vi "MrClean.ProcDestructor.vi"(0 "i ref in":refnum<vi>, 3 "ms timeout (100)":i32=100, 5 "error in (no error)":errorcluster) -> (14 "i ref out":refnum<vi>, 17 "timed out":bool, 19 "error out":errorcluster)   [LabVIEW 2014, in "MrClean.lvlib"]
doc: "This is the counterpart to ProcConstructor and is called befor the \"deactivate\" is called. This can be used to shutdown/deinitialize things."
uses:
  MrClean.lvlib
  CSCore/CSSystem/CoreDefs/CoreDefs.error_type.ctl
  CSCore/CSSystem/CoreLib/CoreLib.string 2 byte array.vi
  CSCore/BaseProcess/BaseProcess.lvlib
  LEBITLib/LEBITLib.lvlib
  CSCore/CSSystem/CSSystemLib/CSSystemLib.lvlib
  CSCore/CSSystem/CoreLib/CoreLib.lvlib
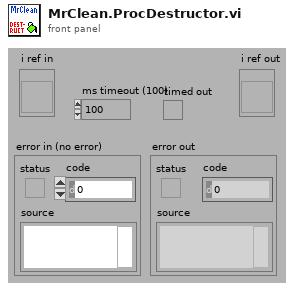
[diagram p1: front panel]
types:
  T1 = typedef "CoreDefs.error_type.ctl" = enum16{"no error", "can't load process", "can't unload process", "process does not exist", "can't install process", "can't remove process", "unknown function", "time out", "can't execute function", "duplicate queue name", "super not found", "caller queue invalid", "can't ping process", "unknown error", "VISA Error", "VISA timeout", "GPIB timeout", "GPIB error", "communication error", "data type mismatch", "can't read data from OPC server", "can't write data to OPC server", "OET error", "function not implemented", "process already exists", "invalid Shared Variable name", "error writing Shared Variable", "error reading Shared Variable", "invalid client name", "corrupt database", "unknown class", "call not authorized", "parameter out of range", "OET timeout: can't get data to modify", "invalid queue name", "requested operation incompatible with current state", "event undefined", "event disabled", "state undefined", "caller is not a friend", "EventBuilder: bad eventID", "EventBuilder: no DAQ devices", "a thread must not stop itself", "UNUSED ELEMENT4", "DiscArchiver: eventData incomplete", "DiscArchiver: eventData does not belong to run", "DiscArchiver: can't open file", "DiscArchiver: can't write to file", "DiscArchiver: available disc space low", "can't acquire semaphore", "error reading data from database", "notifier object is not existing", "can't register process", "can't unregister process", "illegal event type", "object disabled", "object already exists", "can't change state", "Instrument not found", "no connection to remote node", "invalid reference", "N/A", "UNUSED ELEMENT 1", "element not found", "illegal TCP/IP connection detected", "object does not exist", "invalid access ID", "unknown CS system", "invalid privilige", "unsupported data type", "unsupported server type", "IO server already exists", "Shared Variable already exists"}
  T2 = enum16{"simple", "synchronous", "asynchronous", "notification"}
  T3 = typedef "CoreDefs.rawDataType.ctl" = i8[]
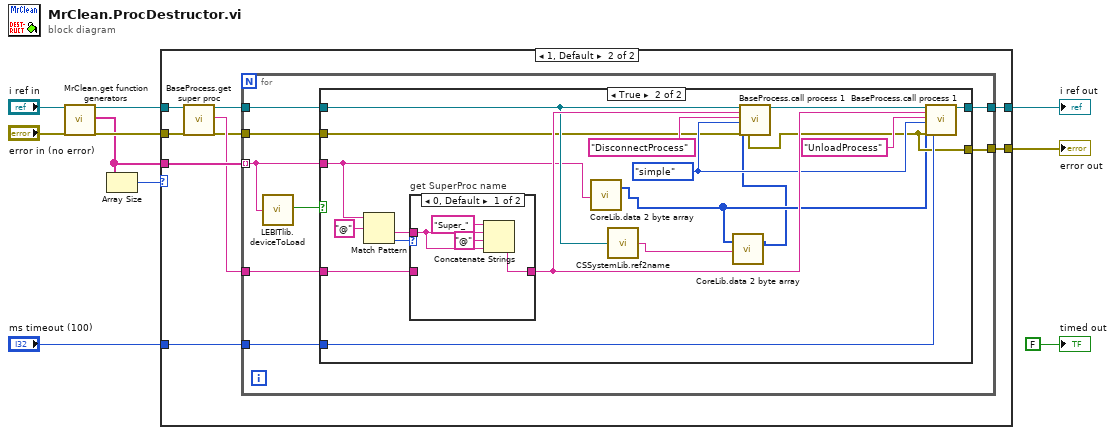
[diagram p0: block diagram]
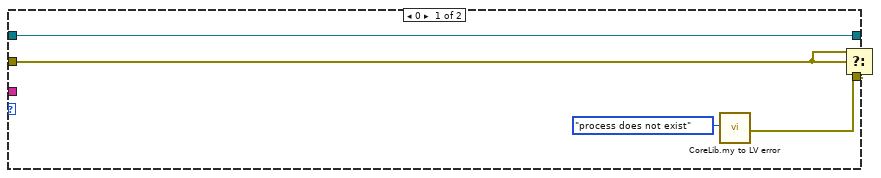
[diagram p2: hidden frame]
diagram:
  n1 = call "MrClean.get function generators.vi"("i ref in"="i ref in", "error in (no error)"="error in (no error)") -> ("i ref out"=w9:refnum<vi>, "function generators"=w7:string[], "error out"=w8:errorcluster)  [unwired: 14 in, 1 out]
  n2 = Array Size(array=w7) -> (size(s)=w10:i32)
  n3 = case shown="1, Default" w10 {
    tunnel: w9 -> [w15 w24]
    tunnel: w8 -> [w13 w23]
    tunnel: w7 -> [_ w21]
    tunnel: "ms timeout (100)" -> [_ w19]
    tunnel: [w14 w16] -> w1
    tunnel: [w15 w18] -> w2
    frame 0 {
      n4 = call "CoreLib.my to LV error.vi"("ErrorTypes"=CoreDefs.error_type."process does not exist") -> ("myErrorCluster"=w12:errorcluster)  [unwired: 17 in, 1 out]
      n5 = Select(t=w13, s=w13, f=w12) -> (s? t:f=w14:errorcluster)
    }
    frame 1, Default {
      n6 = call "BaseProcess.get super proc.vi"("i ref in"=w24, "error in (no error)"=w23) -> ("i ref out"=w22:refnum<vi>, "SuperProc"=w20:string, "error out"=w17:errorcluster)  [unwired: 15 in]
      n7 = for {
        tunnel: w22 -> [w29]
        tunnel: w21 -> [w25] mode=indexing
        tunnel: w20 -> [w32]
        tunnel: w19 -> [w30]
        tunnel: [w31] -> w18
        tunnel: w17 -> [w27]
        tunnel: [w28] -> w16
        n8 = call "LEBITlib.deviceToLoad.vi"("DeviceName"=w25) -> ("DeviceIsToLoad"=w26:bool)
        n9 = case shown="True" w26 {
          tunnel: w32 -> [_ w48]
          tunnel: w25 -> [_ w38]
          tunnel: [w33 w43] -> w31
          tunnel: w30 -> [_ w42]
          tunnel: w29 -> [w33 w40]
          tunnel: w27 -> [w34 w39]
          tunnel: [w34 w39] -> w28
          frame False {
          }
          frame True {
            w45 = T2."simple" ("CallType")
            n10 = Match Pattern(string=w38, regular expression="@") -> (after substring=w49:string, offset past match=w50:i32)  [unwired: 1 in, 2 out]
            n11 = case "get SuperProc name" shown="0, Default" w50 {
              tunnel: w49 -> [w53 _]
              tunnel: w48 -> [_ w56]
              tunnel: [w52 w56] -> w46
              frame 0, Default {
                n12 = Concatenate Strings("Super_" ("string"), w53, "@" ("string"), w53) -> (w52:string)
              }
              frame -1 {
              }
            }
            n13 = call-poly "CoreLib.data 2 byte array.vi"("string"=w38) -> ("byteArray out"=w37:T3)  [unwired: 18 in]
            n14 = call "CSSystemLib.ref2name.vi"("obj refnum"=w40) -> ("name"=w36:string)
            n15 = call-poly "CoreLib.data 2 byte array.vi"("byteArray"=w37, "string"=w36) -> ("byteArray out"=w35:T3)  [unwired: 17 in]
            n16 = call "BaseProcess.call process 1.vi"("i ref in"=w40, "Object"=w46, "Selector"="DisconnectProcess", "CallType"=w45, "Data"=w35, "error in (no error)"=w39) -> ("i ref out"=w41:refnum<vi>)  [unwired: 11 in, 2 out]
            n17 = call "BaseProcess.call process 1.vi"("i ref in"=w41, "Object"=w46, "Selector"="UnloadProcess", "CallType"=w45, "Data"=w37, "error in (no error)"=w39, "timeout (ms)"=w42) -> ("i ref out"=w43:refnum<vi>)  [unwired: 10 in, 2 out]
          }
        }
      }
    }
  }
  "error out" <- w1
  "i ref out" <- w2
  "timed out" <- FALSE ("timed out")
